vi "fgt get sensor Value Ex.vi"(8 "error in (no error)":errorcluster, 11 "sensorIndex":u32) -> (0 "error out":errorcluster, 2 "timeStamp out":i16, 3 "value out":sgl)   [LabVIEW 2016, in "fgt_SDK.lvlib"]
doc: "Read flowrate sensor value and timestamp of selected device. Time stamp is the device internal timer."
uses:
  fgt_SDK.lvlib
  dlls/fgt_SDK_32.dll
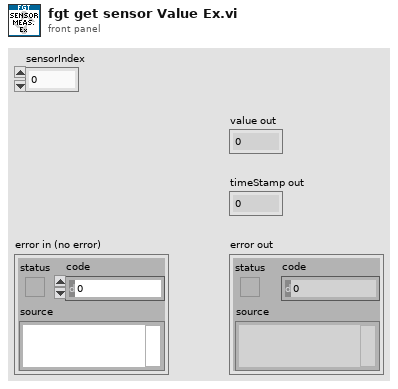
[diagram p1: front panel]
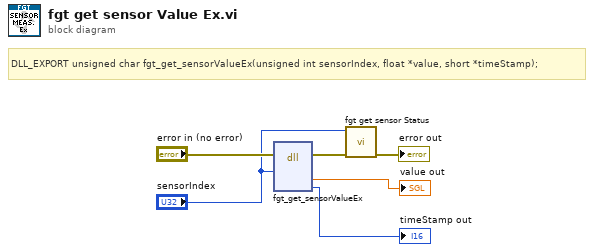
[diagram p0: block diagram]
diagram:
  # "DLL_EXPORT unsigned char fgt_get_sensorValueEx(unsigned int sensorIndex, float *value, short *timeStamp);"
  n1 = dll-call lib="C:/projects/SDK/fgt-sdk-labview/dlls/fgt_SDK_*.*" fn="fgt_get_sensorValueEx"(error in="error in (no error)", "sensorIndex"="sensorIndex") -> (error out=w3:errorcluster, "value"=→"value out":sgl, "timeStamp"=→"timeStamp out":i16)  [unwired: 6 in, 1 out]
  n2 = call "fgt get sensor Status.vi"("error in (no error)"=w3, "pressureIndex"="sensorIndex") -> ("error out"=→"error out":errorcluster)  [unwired: 9 in]
